vi "Frame Import UI.vi"(8 "error in":errorcluster) -> (0 "error out":errorcluster, 1 "Cancelled":bool, 2 "frame map out":map{string, T1}(c390), 3 "Currently Loaded file":path)   [LabVIEW 2020, in "FrameEditor.lvlib"]
doc: "This template is for the Queued Message Handler design pattern.\n\nThe Event Handling Loop generates messages based on user interface actions.\n\nThe Message Handling Loop processes messages generated by the Event Handling Loop, or by other messages. The messages are string values, so new messages can be added easily to the Message Cases case structure in the Message Handling Loop. Each message cluster can also provide an optional value for Message Data, which is a variant that can be converted to whatever message-specific data is required."
uses:
  FrameEditor.lvlib
  controls/frame_record_type.ctl
  <instrlib>/AIM GmbH/_AIM 664/_controls/queue_header_generic.ctl
  controls/UI Data.ctl
  controls/frame_file_entry.ctl
  controls/Type of Payload.ctl
  controls/Payload Record Type.ctl
  <instrlib>/AIM GmbH/_AIM 664/helpers/EthFrameManagement/controls/arinc664_mac_src_info.ctl
  <instrlib>/AIM GmbH/_AIM 664/helpers/EthFrameManagement/controls/arinc664_ip_src_info.ctl
  support/Message Queue/Enqueue Message (Single).vi
  <instrlib>/AIM GmbH/_AIM 664/helpers/EthFrameManagement/Create Payload (Constant).vi
  <instrlib>/AIM GmbH/_AIM 664/helpers/EthFrameManagement/Create Payload (Increment).vi
  <instrlib>/AIM GmbH/_AIM 664/helpers/EthFrameManagement/Create Payload (Random).vi
  <vilib>/Utility/error.llb/Error Cluster From Error Code.vi
  <vilib>/ErrorRing/Error Ring.xnode
  support/Message Queue/Message Queue.lvlib
  support/User Event - Stop/User Event - Stop.lvlib
  <instrlib>/AIM GmbH/_AIM 664/AIM664LV.lvlib
  <instrlib>/AIM GmbH/_AIM 664/helpers/EthFrameManagement/EthFrameManagement.lvlib
panel:
  in  "Frames":i32(listbox)
  out "Destination IP":string
  out "Source MAC":string
  out "Destination MAC":string
  out "Source IP":string
  in  "Partition ID":u8=1
  in  "Interface ID":u8=1 format="%.0b"
  in  "Location ID":u8=1
  in  "Side ID":u8=1
  in  "Domain ID":u8=1
  in  "Increment":u8=1 format="%.0x"
  in  "Start":u8=65 format="%02x"
  in  "Fill Value":u8=10 format="%02x"
  out "option":u32
  in  "Random Payload":bool
  in  "Increment Payload":bool
  in  "Fill Payload":bool
  in  "Bit Length":u16(ring) items=["Byte (8 bits)", "Word (16 bits)", "Long (32 bits)", "Quad (64 bits)"]
  in  "Clear Payload":bool
  in  "Frame ID":string="Frame1"
  in  "Payload Size":u32=17
  in  "Payload":u8[](array[numeric])=[0, 0, 0, 0, 0, 0, 0, 0, 0, 0, 0, 0, 0, 0, 0, 0, 0] format="%02x"
  in  "VL Id":u16=60
  in  "UDP Destination Port":u16=1
  in  "UDP Source Port":u16=1
  in  "Header Information":T3={"Inter Frame Gap"=0, "Packet Group Wait Time"=10000, "Payload Buffer Mode"=0, "Payload Generation Mode"=0, "Preamble Count"=7, "Skew"=0, "Net Select"=4, "Frame Start Mode"=1, "Physical Error Injection"=0, "Sequence Number Init"=65535, "Sequence Number Offset"=65535} {"Net Select" items=["FDX_TX_FRAME_DLY_A"=0, "FDX_TX_FRAME_DLY_B"=1, "FDX_TX_FRAME_BOTH "=3, "FDX_TX_FRAME_ONLY_A"=4, "FDX_TX_FRAME_ONLY_B "=5]; "Frame Start Mode" items=["FDX_TX_FRAME_START_IFG", "FDX_TX_FRAME_START_PGWT", "FDX_TX_FRAME_START_TRG"]; "Physical Error Injection" items=["FDX_TX_FRAME_ERR_OFF"=0, "FDX_TX_FRAME_ERR_CRC"=1, "FDX_TX_FRAME_ERR_ALI"=2, "FDX_TX_FRAME_ERR_PRE"=4, "FDX_TX_FRAME_ERR_PHY"=8]; "Sequence Number Init" items=["FDX_TX_FRAME_SEQ_INIT_AUTO"=65535]; "Sequence Number Offset" items=["FDX_TX_FRAME_SEQ_OFFS_AUTO "=65535]; "Payload Generation Mode" items=["FDX_TX_FRAME_PGM_USER"=0, "FDX_TX_FRAME_PGM_IP_PART"=1, "FDX_TX_FRAME_PGM_IP_FULL"=2, "FDX_TX_FRAME_PGM_IP_PART_TT"=10, "FDX_TX_FRAME_PGM_IP_FULL_TT"=20]; "Payload Buffer Mode" items=["FDX_TX_FRAME_PBM_STD", "FDX_TX_FRAME_PBM_MAC", "FDX_TX_FRAME_PBM_UDP"]}
  out "Payload Entry":string[][](table)
  out "Display Message":string
  in  "Convert":bool
  in  "Cancel":bool
  in  "Load":bool
  in  "Save":bool
  in  "Remove":bool
  in  "Add":bool
  in  "Exit":bool
  # "Auto-generate Payload"
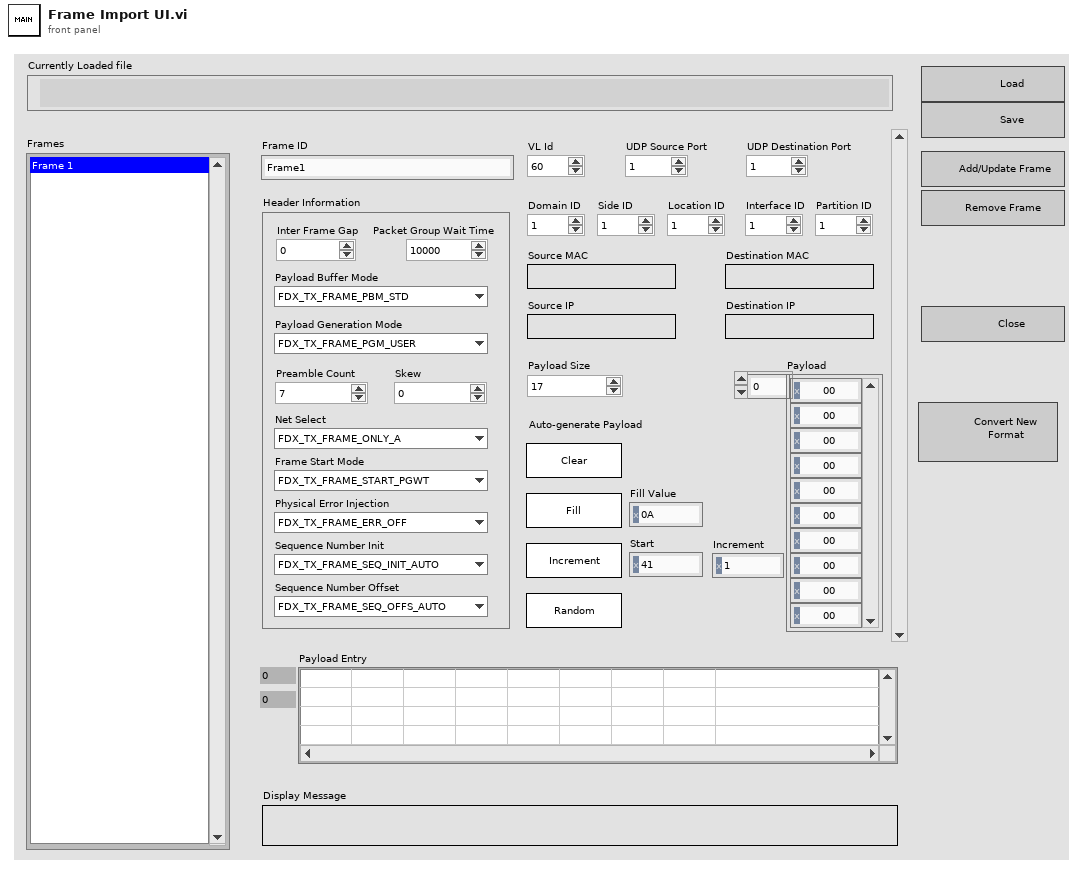
[diagram p1: front panel]
types:
  T1 = typedef "frame_record_type.ctl" = cluster{"HeaderInfo":T2, "Data":u8[]}
  T2 = typedef "AIM664LV.lvlib/queue_header_generic.ctl" = cluster{"InterFrameGap":u32, "PacketGroupWaitTime":u32, "PayloadBufferMode":u8, "PayloadGenerationMode":u8, "PreambleCount":u8, "Skew":u32, "NetSelect":u8, "FrameStartMode":u8, "PhysErrorInjection":u32, "SequenceNumberInit":u16, "SequenceNumberOffset":u16}
  T3 = cluster{"Inter Frame Gap":u32, "Packet Group Wait Time":u32, "Payload Buffer Mode":u8, "Payload Generation Mode":u8, "Preamble Count":u8, "Skew":u32, "Net Select":u8, "Frame Start Mode":u8, "Physical Error Injection":u32, "Sequence Number Init":u16, "Sequence Number Offset":u16}
  T4 = typedef "UI Data.ctl" = cluster{"changesPending":bool, "String <Replace Me>":string, "Numeric <Replace Me>":dbl, "Add":refnum<vi>, "Remove":refnum<vi>, "Data Display Ref":refnum<vi>, "Exit Button Ref":refnum<vi>, "Load":refnum<vi>, "Save":refnum<vi>, "Payload ID":refnum<vi>, "Type of Frame":refnum<vi>}
  T5 = typedef "FrameEditor.lvlib/Message Queue.lvlib/All Message Queues.ctl" = cluster{"UI":refnum<queue>}
  T6 = typedef "frame_file_entry.ctl" = cluster{"key":string, "value":T1}
  T7 = enum16{"open", "replace", "create", "open or create", "replace or create", "replace or create with confirmation"}
  T8 = typedef "Payload Record Type.ctl" = cluster{"Data":u8[], "Type of Frame":T9}
  T9 = typedef "Type of Payload.ctl" = u16
  T10 = typedef "EthFrameManagement.lvlib/arinc664_ip_src_info.ctl" = cluster{"domainID":u8, "sideID":u8, "locationID":u8, "partitionID":u8}
  T11 = typedef "EthFrameManagement.lvlib/arinc664_mac_src_info.ctl" = cluster{"domainID":u8, "sideID":u8, "locationID":u8, "interfaceID":u8}
  T12 = cluster{"Domain ID":u8, "Side ID":u8, "Location ID":u8, "Interface ID":u8, "Partition ID":u8}
  T13 = typedef "AIM664LV.lvlib/queue_data_full.ctl" = cluster{"domainID":u8, "sideID":u8, "locationID":u8, "interfaceID":u8, "partitionID":u8}
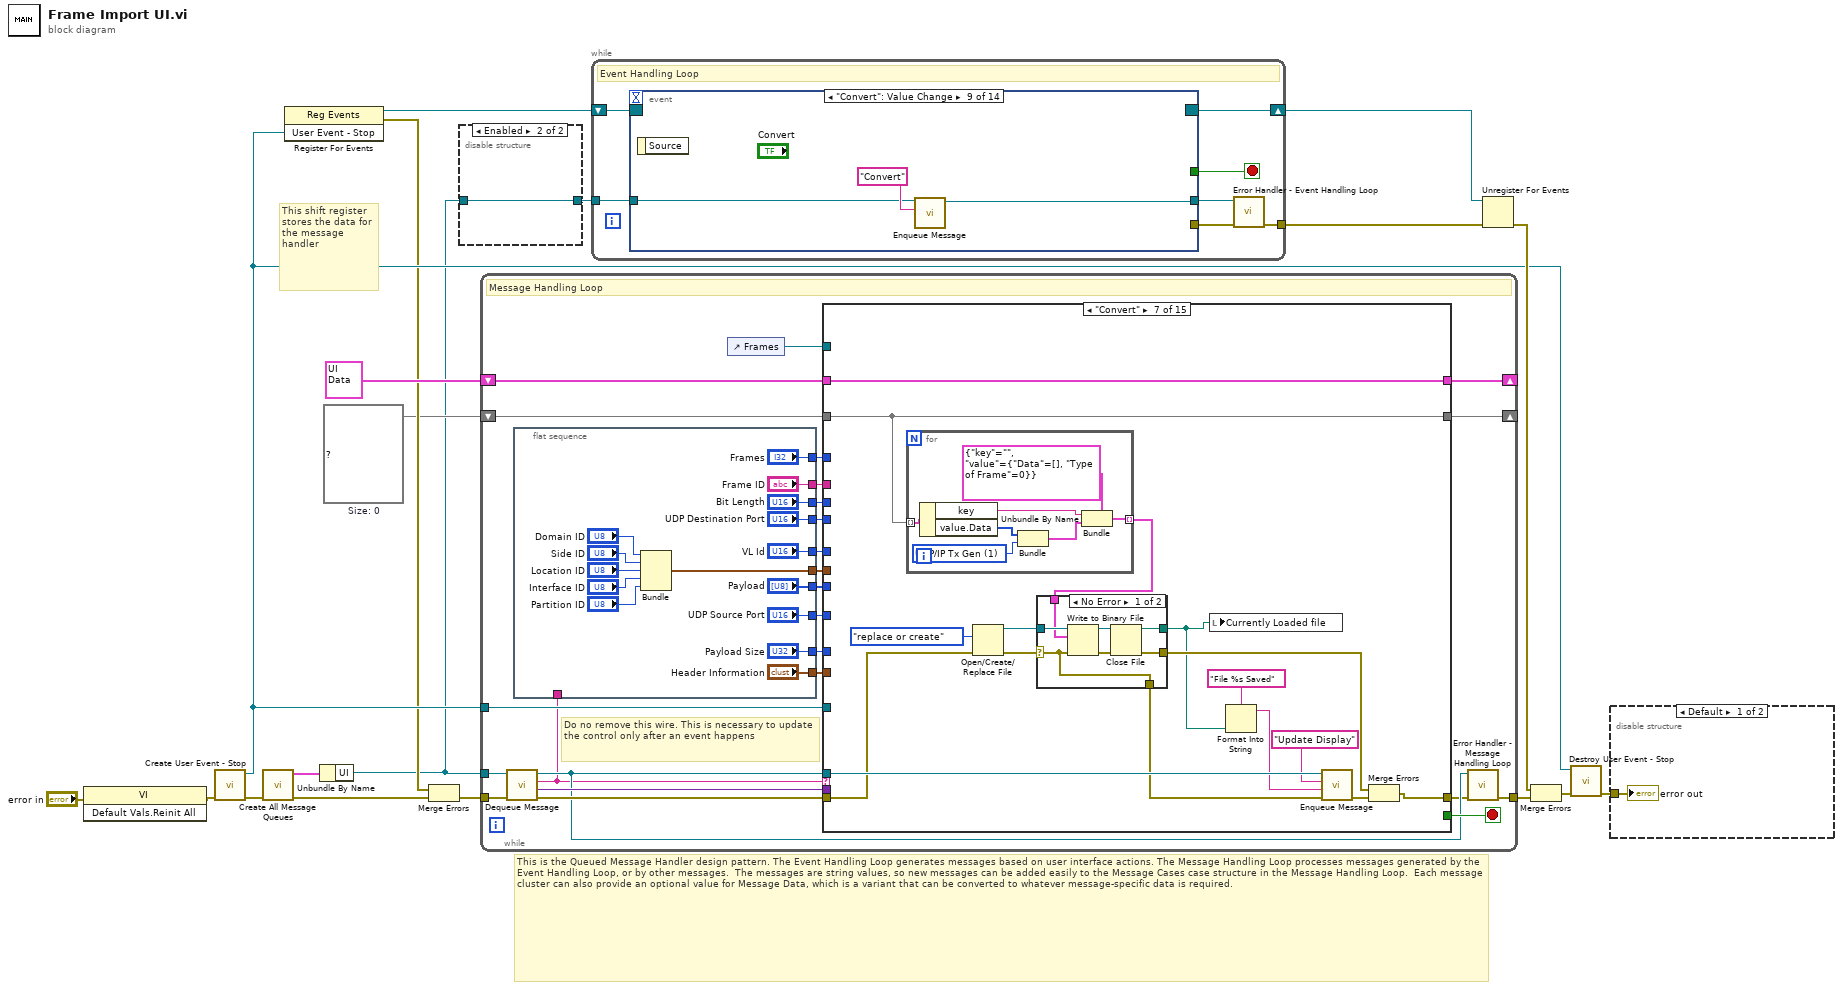
[diagram p0: block diagram]
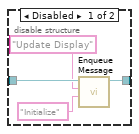
[diagram p2: hidden frame]
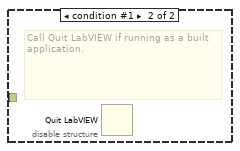
[diagram p3: hidden frame]
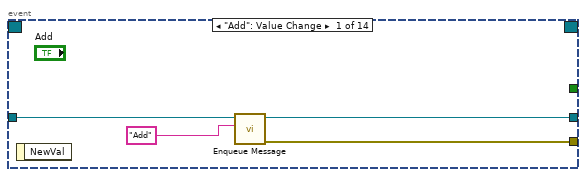
[diagram p4: hidden frame]
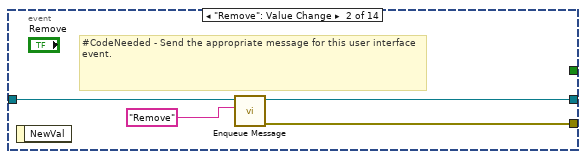
[diagram p5: hidden frame]
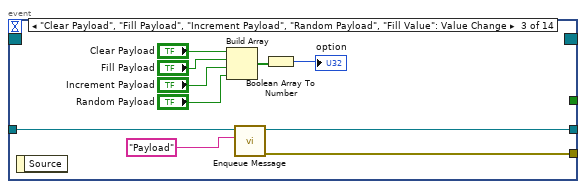
[diagram p6: hidden frame]
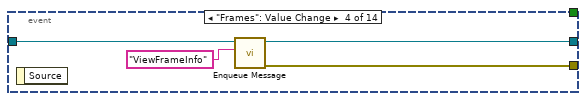
[diagram p7: hidden frame]
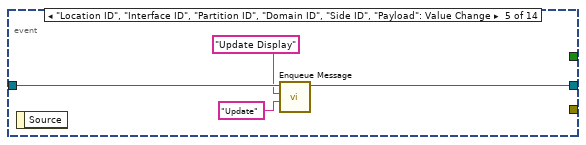
[diagram p8: hidden frame]
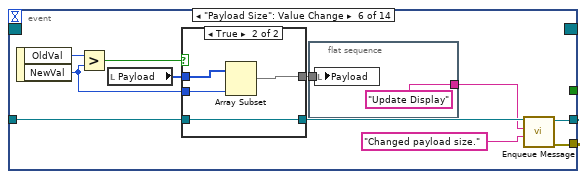
[diagram p9: hidden frame]
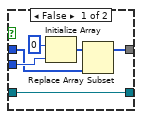
[diagram p10: hidden frame]
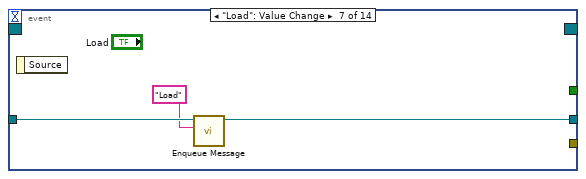
[diagram p11: hidden frame]
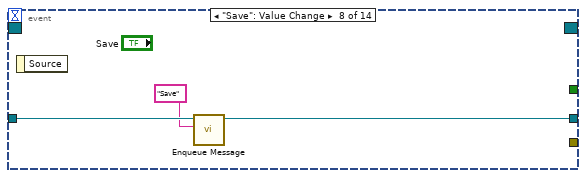
[diagram p12: hidden frame]
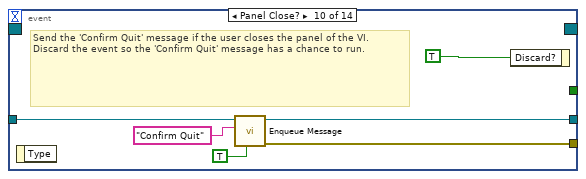
[diagram p13: hidden frame]
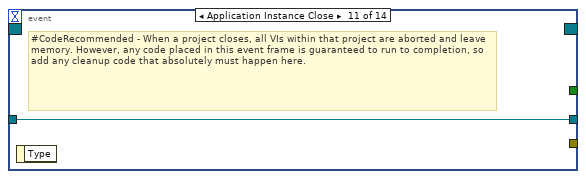
[diagram p14: hidden frame]
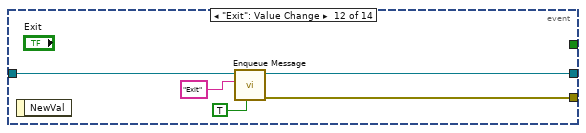
[diagram p15: hidden frame]
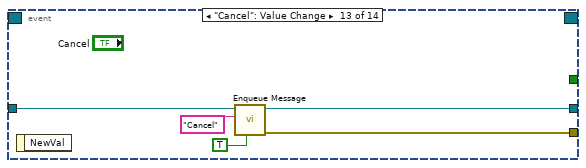
[diagram p16: hidden frame]
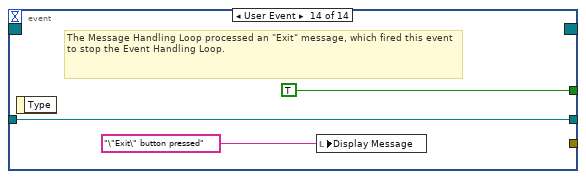
[diagram p17: hidden frame]
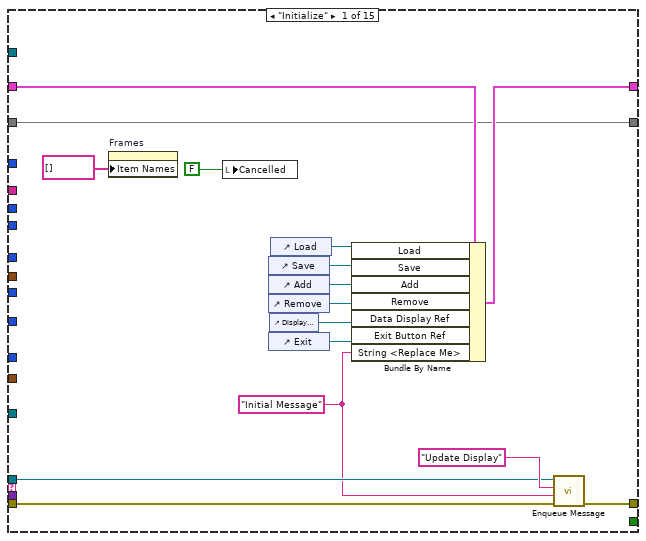
[diagram p18: hidden frame]
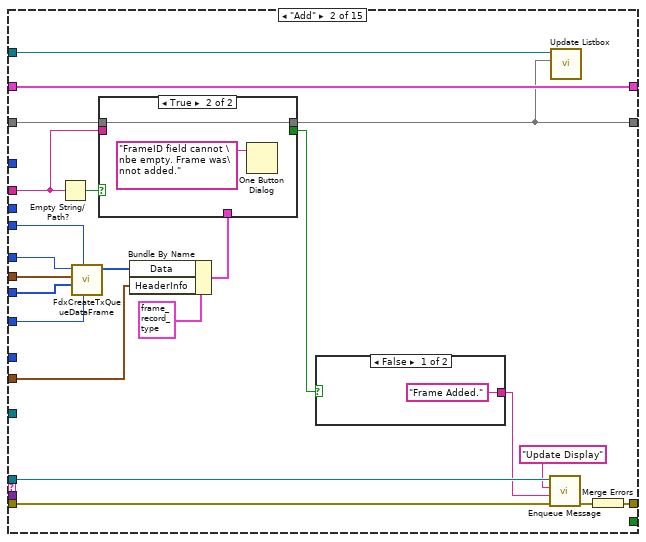
[diagram p19: hidden frame]
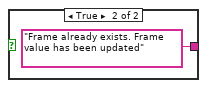
[diagram p20: hidden frame]
diagram:
  w5 = map{string, T1} {}  # Size: 0
  # "This is the Queued Message Handler design pattern. The Event Handling Loop generates messages based on user interface actions. The Message Handling Loop processes messages generated by the Event Handling Loop, or by other messages.  The messages are string values, so new messages can be added easily to the Message Cases case structure in the Message Handling Loop.  Each message cluster can also provide an optional value for Message Data, which is a variant that can be converted to whatever message-specific data is required."
  # "This shift register stores the data for the message handler"
  n1 = invoke class="VI" method="Default Vals.Reinit All"(error in="error in") -> (error out=w2:errorcluster)  [unwired: 2 in, 2 out]
  n2 = call "Create User Event - Stop.vi"("error in (no error)"=w2) -> ("error out"=w16:errorcluster, "User Event - Stop"=w8:refnum<user-event>)  [unwired: 9 in]
  n3 = call "Create All Message Queues.vi"("error in (no error)"=w16) -> ("error out"=w19:errorcluster, "Message Queues out"=w18:T5)  [unwired: 9 in]
  n4 = register-events(w8) -> (reference out=w9:refnum<event-registration>, error out=w6:errorcluster)  [unwired: 2 in]
  n5 = Unbundle By Name(w18) -> ("UI"=w4:refnum<queue>)
  n6 = Merge Errors(w6, w19) -> (w7:errorcluster)
  n7 = disable-structure shown="Enabled" {
    disable-tunnel: w4 -> [w23 w24]
    disable-tunnel: [w22 w24] -> w3
    frame Disabled {
      n8 = call-poly "Enqueue Message.vi"("Message Data"="Initialize" ("Message"), "Message"="Update Display", "Message Queue"=w23) -> ("dup Message Queue"=w22:refnum<queue>)  [unwired: 7 in, 1 out]
    }
    frame Enabled {
    }
  }
  n9 = while {
    tunnel: w4 -> [w42]
    shift-right: [w48] -> _
    shift-left: T4 {"changesPending"=FALSE, "String <Replace Me>"="", "Numeric <Replace Me>"=0.0, "Add"=refnum, "Remove"=refnum, "Data Display Ref"=refnum, "Exit Button Ref"=refnum, "Load"=refnum, "Save"=refnum, "Payload ID"=refnum, "Type of Frame"=refnum} ("Data Cluster") -> [w49]
    tunnel: w8 -> [w46]
    tunnel: w7 -> [w45]
    tunnel: [w40] -> w17
    shift-right: [w29] -> _
    shift-left: w5 -> [w31]
    stop <- w47 stop-if-true
    # "Do no remove this wire. This is necessary to update the control only after an event happens"
    # "Message Handling Loop"
    n10 = call "Dequeue Message.vi"("error in (no error)"=w45, "Message Queue"=w42) -> ("error out"=w44:errorcluster, "Message Data"=w43:variant, "Message"=w25:string, "dup Message Queue"=w41:refnum<queue>)  [unwired: 6 in]
    n11 = flat-sequence {
      tunnel: ["Payload Size"] -> w38
      tunnel: [w63] -> w37
      tunnel: ["VL Id"] -> w36
      tunnel: ["UDP Source Port"] -> w35
      tunnel: ["UDP Destination Port"] -> w34
      tunnel: ["Payload"] -> w33
      tunnel: ["Header Information"] -> w32
      tunnel: ["Frame ID"] -> w30
      tunnel: ["Frames"] -> w28
      tunnel: ["Bit Length"] -> w26
      tunnel: w25 -> [_]
      frame #0 {
        n12 = Bundle("Domain ID"="Domain ID", "Side ID"="Side ID", "Location ID"="Location ID", "Interface ID"="Interface ID", "Partition ID"="Partition ID") -> (w63:T12)  [unwired: 1 in]
      }
    }
    n13 = control-ref of="Frames"() -> (w27:refnum<vi>)
    n14 = case "Message Cases" shown="\"Convert\"" w25 {
      selector: w25 -> [_ _ _ _ _ _ _ _ _ _ _ _ _ _ w395]
      tunnel: w41 -> [w71 w98 w123 w162 w178 w213 w244 _ _ w328 _ w339 w380 w393 _]
      tunnel: w44 -> [w79 w100 w120 w164 w180 w211 w242 w302 w324 w332 w336 w342 w373 w386 _]
      tunnel: [w80 w101 w125 w165 w181 w215 w246 w303 w318 w330 w334 w347 w376 w389 w396] -> w39
      tunnel: w49 -> [w78 w102 w126 w166 w182 w216 w247 w304 w323 w331 w335 w348 w379 w392 w397]
      tunnel: [w77 w102 w126 w166 w182 w216 w247 w304 w323 w331 w335 w348 w379 w392 w397] -> w48
      tunnel: [_ _ _ _ _ _ _ _ _ _ _ _ TRUE TRUE _] -> w47
      tunnel: w43 -> [_ _ _ _ _ _ _ w301 w322 _ _ _ w370 w383 _]
      tunnel: w46 -> [_ _ _ _ _ _ _ _ _ _ _ _ w375 w388 _]
      tunnel: w38 -> [_ _ _ _ _ _ _ _ _ _ _ w345 _ _ _]
      tunnel: w37 -> [_ w95 _ _ _ _ _ w284 _ _ _ _ _ _ _]
      tunnel: w36 -> [_ w96 _ _ _ _ _ w285 _ _ _ _ _ _ _]
      tunnel: w35 -> [_ w92 _ _ _ _ _ _ _ _ _ _ _ _ _]
      tunnel: w34 -> [_ w94 _ _ _ _ _ _ _ _ _ _ _ _ _]
      tunnel: w33 -> [_ w93 _ _ _ _ _ w266 _ _ _ _ _ _ _]
      tunnel: w32 -> [_ w90 _ _ _ _ _ _ _ _ _ _ _ _ _]
      tunnel: w31 -> [w67 w85 w112 w159 w174 w210 w241 w269 w317 w325 w333 w346 w369 w382 w394]
      tunnel: w30 -> [_ w86 _ _ _ _ _ _ _ _ _ _ _ _ _]
      tunnel: [w67 w84 w117 w156 w174 w210 w241 w269 w317 w325 w333 w346 w369 w382 w394] -> w29
      tunnel: w28 -> [_ _ _ w152 w176 _ _ _ _ _ _ _ _ _ _]
      tunnel: w27 -> [_ w88 w121 w157 w175 _ _ w268 _ _ _ _ _ _ _]
      tunnel: w26 -> [_ _ _ _ _ _ _ w297 _ _ _ w344 _ _ _]
      frame "Initialize" {
        w70 = "Initial Message" ("Initial Message")
        # "Initialize - All initialization work should take place in this message, since other loops can potentially enqueue messages that execute immediately after this one."
        n15 = property on="Frames" class="LstBox (strict)"("Item Names"=string[] []) -> ()  [unwired: 2 in, 2 out]
        n16 = local write "Cancelled"(FALSE ("Cancel")) -> ()
        n17 = control-ref of="Save"() -> (w68:refnum<vi>)
        n18 = control-ref of="Add"() -> (w76:refnum<vi>)
        n19 = control-ref of="Remove"() -> (w75:refnum<vi>)
        n20 = control-ref of="Exit"() -> (w73:refnum<vi>)
        n21 = control-ref of="Display Message"() -> (w74:refnum<vi>)
        n22 = control-ref of="Load"() -> (w69:refnum<vi>)
        n23 = Bundle By Name(cluster=w78, "Load"=w69, "Save"=w68, "Add"=w76, "Remove"=w75, "Data Display Ref"=w74, "Exit Button Ref"=w73, "String <Replace Me>"=w70) -> (w77:T4)
        n24 = call-poly "Enqueue Message.vi"("error in (no error)"=w79, "Message Data"=w70, "Message"="Update Display", "Message Queue"=w71) -> ("error out"=w80:errorcluster)  [unwired: 6 in, 1 out]
      }
      frame "Add" {
        # "Something - Replace this message with functionality for your own application."
        n25 = Empty String/Path?(string/path=w86) -> (empty?=w87:bool)
        n26 = call <instrlib>:"FdxCreateTxQueueDataFrame.vi"("UDPsrcPort"=w92, "UDPdstPort"=w94, "Payload"=w93, "afdx configuration"=w95, "VL Id"=w96) -> ("Frame"=w89:u8[])  [unwired: 4 in, 2 out]
        n27 = Bundle By Name(cluster=T1 {"HeaderInfo"={"InterFrameGap"=0, "PacketGroupWaitTime"=10000, "PayloadBufferMode"=0, "PayloadGenerationMode"=0, "PreambleCount"=7, "Skew"=0, "NetSelect"=4, "FrameStartMode"=1, "PhysErrorInjection"=0, "SequenceNumberInit"=65535, "SequenceNumberOffset"=65535}, "Data"=[10]}, "Data"=w89, "HeaderInfo"=w90) -> (w83:T1)
        n28 = case shown="True" w87 {
          tunnel: w86 -> [w108 _]
          tunnel: w85 -> [w109 w110]
          tunnel: [w107 w110] -> w84
          tunnel: w83 -> [w106 _]
          tunnel: [w105 _] -> w82
          frame False {
            n29 = Insert Into Map(map in=w109, key=w108, value=w106) -> (map out=w107:map{string, T1}, key already included?=w105:bool)  [unwired: 1 out]
          }
          frame True {
            n30 = One Button Dialog(message="FrameID field cannot \nbe empty. Frame was\nnot added.") -> ()  [unwired: 1 in, 1 out]
          }
        }
        n31 = case shown="False" w82 {
          tunnel: ["Frame Added." ("format string") "Frame already exists. Frame value has been updated" ("format string")] -> w81
          frame False {
          }
          frame True {
          }
        }
        n32 = call-poly "Enqueue Message.vi"("error in (no error)"=w100, "Message Data"=w81, "Message"="Update Display", "Message Queue"=w98) -> ("error out"=w99:errorcluster)  [unwired: 6 in, 1 out]
        n33 = call "Update Listbox.vi"("frame map"=w84, "ListBox ref"=w88) -> ()  [unwired: 10 in]
        n34 = Merge Errors(w99) -> (w101:errorcluster)
      }
      frame "Load" {
        # "Something - Replace this message with functionality for your own application."
        n35 = Open/Create/Replace File(error in=w120) -> (refnum out=w118:refnum<file>, error out=w113:errorcluster)  [unwired: 5 in, 1 out]
        n36 = case shown="No Error" w113 {
          tunnel: w121 -> [w139 _]
          tunnel: [w128 _] -> w119
          tunnel: w118 -> [w138 _]
          tunnel: [w135 w151] -> w117
          tunnel: [w134 path "" ("path")] -> w115
          tunnel: w113 -> [w133 _]
          tunnel: ["File %s Loaded" ("format string") "Load Cancelled." ("format string")] -> w114
          tunnel: w112 -> [w127 w151]
          frame No Error {
            w137 = map{string, T1} {}  # Size: 0
            n37 = Read from Binary File(5:T6[] [] ("cluster"), 8:w133, 11:w138) -> (0:w131:errorcluster, 2:w136:T6[], 3:w130:refnum<file>)  [unwired: 3 in, 1 out]
            n38 = Close File(refnum=w130, error in=w131) -> (path=w134:path, error out=w128:errorcluster)
            n39 = case shown="No Error" w128 {
              tunnel: w137 -> [w142 _]
              tunnel: w136 -> [w141 _]
              tunnel: [w140 w148] -> w135
              tunnel: w127 -> [_ w148]
              frame No Error {
                n40 = for {
                  shift-right: [w146] -> w140
                  shift-left: w142 -> [w147]
                  tunnel: w141 -> [w145] mode=indexing
                  n41 = Unbundle By Name(w145) -> ("key"=w144:string, "value"=w143:T1)
                  n42 = Insert Into Map(map in=w147, key=w144, value=w143) -> (map out=w146:map{string, T1})  [unwired: 2 out]
                }
              }
              frame Error {
                # "Any error, we keep what we \nhad before."
              }
            }
            n43 = local write "Currently Loaded file"(w134) -> ()
            n44 = call "Update Listbox.vi"("frame map"=w135, "ListBox ref"=w139) -> ()  [unwired: 10 in]
          }
          frame Error {
          }
        }
        n45 = Format Into String(format string=w114, w115) -> (resulting string=w116:string)  [unwired: 2 in, 1 out]
        n46 = call-poly "Enqueue Message.vi"("error in (no error)"=w120, "Message Data"=w116, "Message"="Update Display", "Message Queue"=w123) -> ("error out"=w124:errorcluster)  [unwired: 6 in, 1 out]
        n47 = Merge Errors(w119, w124) -> (w125:errorcluster)
      }
      frame "Remove" {
        # "Something Else - Replace this message with functionality for your own application."
        n48 = invoke on="Frame ID" class="Str" method="Reinit To Default"() -> ()  [unwired: 3 in, 3 out]
        n49 = invoke on="UDP Destination Port" class="DigNum (strict)" method="Reinit To Default"() -> ()  [unwired: 3 in, 3 out]
        n50 = invoke on="VL Id" class="DigNum (strict)" method="Reinit To Default"() -> ()  [unwired: 3 in, 3 out]
        n51 = property on="Frames" class="LstBox (strict)"() -> ("Item Names"=w160:string[])  [unwired: 2 in, 2 out]
        n52 = Equal?(x=w152, y=-1) -> (x = y?=w154:bool)
        n53 = Index Array(array=w160, index=w152) -> (element=w158:string)
        n54 = case shown="False" w154 {
          tunnel: ["Frame removed." ("format string") "Frame was not selected, so no Frames were removed." ("format string")] -> w153
          frame False {
          }
          frame True {
          }
        }
        n55 = invoke on="UDP Source Port" class="DigNum (strict)" method="Reinit To Default"() -> ()  [unwired: 3 in, 3 out]
        n56 = invoke on="Payload" class="Arr (strict)" method="Reinit To Default"() -> ()  [unwired: 3 in, 3 out]
        n57 = invoke on="Payload Size" class="DigNum (strict)" method="Reinit To Default"() -> ()  [unwired: 3 in, 3 out]
        n58 = invoke on="Header Information" class="Clust (strict)" method="Reinit To Default"() -> ()  [unwired: 3 in, 3 out]
        n59 = Remove From Map(10:w158, 11:w159) -> (3:w156:map{string, T1})  [unwired: 2 out]
        n60 = call "Update Listbox.vi"("frame map"=w156, "ListBox ref"=w157) -> ()  [unwired: 10 in]
        n61 = call-poly "Enqueue Message.vi"("error in (no error)"=w164, "Message Data"=w153, "Message"="Update Display", "Message Queue"=w162) -> ("error out"=w163:errorcluster)  [unwired: 6 in, 1 out]
        n62 = Merge Errors(w163) -> (w165:errorcluster)
      }
      frame "ViewFrameInfo" {
        # "Something Else - Replace this message with functionality for your own application."
        n63 = property on="Frames" class="LstBox (strict)"() -> ("Item Names"=w177:string[])  [unwired: 2 in, 2 out]
        n64 = Index Array(array=w177, index=w176) -> (element=w169:string)
        n65 = Look In Map(map=w174, key=w169) -> (key not found?=w173:bool, value=w172:T1)  [unwired: 1 in]
        n66 = case shown="False" w173 {
          tunnel: w172 -> [w199 _]
          tunnel: [w197 "Frame not found"] -> w170
          tunnel: w169 -> [w190 _]
          frame False {
            n67 = Unbundle By Name(w199) -> ("HeaderInfo"=w196:T2, "Data"=w194:u8[])
            n68 = local write "Frame ID"(w190) -> ()
            n69 = local write "Header Information"(w196) -> ()
            n70 = call "Parse Raw Frame.vi"("Data"=w194, "HeaderInfo"=w196) -> ("UDPsrcPort"=w191:u16, "UDPdstPort"=w192:u16, "VL Id"=w193:u16, "Payload"=w184:u8[], "Frame Configuration"=w195:T13)  [unwired: 5 in]
            n71 = Format Into String(format string="Frame %s displayed", w190) -> (resulting string=w197:string)  [unwired: 2 in, 1 out]
            n72 = Unbundle(w195) -> ("domainID"=w189:u8, "sideID"=w185:u8, "locationID"=w188:u8, "interfaceID"=w186:u8, "partitionID"=w187:u8)
            n73 = Array Size(array=w184) -> (size(s)=w183:i32)
            n74 = local write "UDP Destination Port"(w192) -> ()
            n75 = local write "UDP Source Port"(w191) -> ()
            n76 = local write "Payload Size"(w183) -> ()
            n77 = local write "Location ID"(w188) -> ()
            n78 = local write "Interface ID"(w186) -> ()
            n79 = local write "Partition ID"(w187) -> ()
            n80 = local write "Domain ID"(w189) -> ()
            n81 = local write "Payload"(w184) -> ()
            n82 = local write "Side ID"(w185) -> ()
            n83 = local write "VL Id"(w193) -> ()
          }
          frame True {
          }
        }
        n84 = call "Update Listbox.vi"("frame map"=w174, "ListBox ref"=w175) -> ()  [unwired: 10 in]
        n85 = call-poly "Enqueue Message.vi"("error in (no error)"=w180, "Message Data"=w170, "Message"="Update Display", "Message Queue"=w178) -> ("error out"=w179:errorcluster)  [unwired: 6 in, 1 out]
        n86 = Merge Errors(w179) -> (w181:errorcluster)
      }
      frame "Save" {
        # "Something Else - Replace this message with functionality for your own application."
        n87 = for {
          tunnel: w210 -> [w231] mode=indexing
          tunnel: [w228] -> w207 mode=indexing
          n88 = Unbundle By Name(w231) -> ("key"=w230:string, "value"=w229:T1)
          n89 = Bundle(cluster=T6 {"key"="", "value"={"HeaderInfo"={"InterFrameGap"=0, "PacketGroupWaitTime"=0, "PayloadBufferMode"=0, "PayloadGenerationMode"=0, "PreambleCount"=0, "Skew"=0, "NetSelect"=0, "FrameStartMode"=0, "PhysErrorInjection"=0, "SequenceNumberInit"=0, "SequenceNumberOffset"=0}, "Data"=[]}}, "key"=w230, "value"=w229) -> (w228:T6)
        }
        n90 = Open/Create/Replace File(error in=w211, operation (0:open)=T7."replace or create") -> (refnum out=w209:refnum<file>, error out=w202:errorcluster)  [unwired: 4 in, 1 out]
        n91 = case shown="No Error" w202 {
          selector: w202 -> [w217 w225]
          tunnel: w209 -> [w223 _]
          tunnel: [w220 w224] -> w208
          tunnel: w207 -> [w219 _]
          tunnel: [w218 _] -> w204
          tunnel: [w217 w224] -> w201
          frame No Error {
            n92 = Write to Binary File(file (use dialog)=w223, data=w219, error in=w217) -> (refnum out=w221:refnum<file>, error out=w222:errorcluster)  [unwired: 3 in, 1 out]
            n93 = Close File(refnum=w221, error in=w222) -> (path=w218:path, error out=w220:errorcluster)
          }
          frame Error {
            n94 = call <vilib>:"Clear Errors.vi"("error in (no error)"=w225, "specific error code to clear (0: all)"=43) -> ("error out"=w224:errorcluster)  [unwired: 4 in, 1 out]
          }
        }
        "Currently Loaded file" <- w204
        n95 = Format Into String(format string="File %s Saved", w204) -> (resulting string=w206:string)  [unwired: 2 in, 1 out]
        n96 = call-poly "Enqueue Message.vi"("error in (no error)"=w201, "Message Data"=w206, "Message"="Update Display", "Message Queue"=w213) -> ("error out"=w214:errorcluster)  [unwired: 6 in, 1 out]
        n97 = Merge Errors(w208, w214) -> (w215:errorcluster)
      }
      frame "Convert" {
        # "Something Else - Replace this message with functionality for your own application."
        n98 = for {
          tunnel: w241 -> [w264] mode=indexing
          tunnel: [w259] -> w238 mode=indexing
          w263 = T9 1 items=["Raw Frame", "UDP/IP Tx Gen", "Tx UDP"] ("Type of Frame")
          n99 = Unbundle By Name(w264) -> ("key"=w260:string, "value.Data"=w262:u8[])
          n100 = Bundle("Data"=w262, "Type of Frame"=w263) -> (w261:cluster{"Data":u8[], "Type of Frame":T9})  [unwired: 1 in]
          n101 = Bundle(cluster=cluster{"key":string, "value":T8} {"key"="", "value"={"Data"=[], "Type of Frame"=0}}, "key"=w260, "value"=w261) -> (w259:cluster{"key":string, "value":T8})
        }
        n102 = Open/Create/Replace File(error in=w242, operation (0:open)=T7."replace or create") -> (refnum out=w240:refnum<file>, error out=w234:errorcluster)  [unwired: 4 in, 1 out]
        n103 = case shown="No Error" w234 {
          selector: w234 -> [w248 w256]
          tunnel: w240 -> [w254 _]
          tunnel: [w251 w255] -> w239
          tunnel: w238 -> [w250 _]
          tunnel: [w249 _] -> w232
          tunnel: [w248 w255] -> w233
          frame No Error {
            n104 = Write to Binary File(file (use dialog)=w254, data=w250, error in=w248) -> (refnum out=w252:refnum<file>, error out=w253:errorcluster)  [unwired: 3 in, 1 out]
            n105 = Close File(refnum=w252, error in=w253) -> (path=w249:path, error out=w251:errorcluster)
          }
          frame Error {
            n106 = call <vilib>:"Clear Errors.vi"("error in (no error)"=w256, "specific error code to clear (0: all)"=43) -> ("error out"=w255:errorcluster)  [unwired: 4 in, 1 out]
          }
        }
        n107 = local write "Currently Loaded file"(w232) -> ()
        n108 = Format Into String(format string="File %s Saved", w232) -> (resulting string=w237:string)  [unwired: 2 in, 1 out]
        n109 = call-poly "Enqueue Message.vi"("error in (no error)"=w233, "Message Data"=w237, "Message"="Update Display", "Message Queue"=w244) -> ("error out"=w245:errorcluster)  [unwired: 6 in, 1 out]
        n110 = Merge Errors(w239, w245) -> (w246:errorcluster)
      }
      frame "Update Display" {
        # "Update Display - Convert the message data to a string to display in the Data Display indicator."
        n111 = Increment(x=w297) -> (x+1=w295:u16)
        n112 = Multiply(x=w295, y=u16 8) -> (x*y=w265:u16)
        n113 = Variant To Data(error in=w302, type="", Variant=w301) -> (data=→"Display Message":string, error out=w299:errorcluster)
        n114 = call "Convert Non-visible Char to Visible Char.vi"("bytes per row"=w265, "data"=w266) -> ("data table"=→"Payload Entry":string[][])  [unwired: 7 in, 2 out]
        n115 = Unbundle By Name(w284) -> ("Domain ID"=w289:u8, "Side ID"=w288:u8, "Location ID"=w287:u8, "Interface ID"=w292:u8, "Partition ID"=w286:u8)
        n116 = Bundle By Name(cluster=T11 {"domainID"=0, "sideID"=0, "locationID"=0, "interfaceID"=1} ("Source Info"), "domainID"=w289, "sideID"=w288, "locationID"=w287, "interfaceID"=w292) -> (w293:T11)
        n117 = Bundle By Name(cluster=T10 {"domainID"=0, "sideID"=0, "locationID"=0, "partitionID"=1} ("Source Info"), "domainID"=w289, "sideID"=w288, "locationID"=w287, "partitionID"=w286) -> (w290:T10)
        n118 = call <instrlib>:"Create ARINC-664 IP (Dest).vi"("VL"=w285) -> ("ip string"=→"Destination IP":string)  [unwired: 8 in, 2 out]
        n119 = call <instrlib>:"Create ARINC-664 MAC (Dest).vi"("VL Id"=w285) -> ("MAC-src"=w279:u8[])  [unwired: 9 in, 1 out]
        n120 = for {
          tunnel: w279 -> [w310] mode=indexing
          shift-right: [w306] -> w270
          shift-left: "" -> [w305]
          n121 = Number To Hexadecimal String(1:i16 2 ("width (-)"), 2:w310) -> (0:w308:string)
          n122 = Concatenate Strings(w305, w308, ":" ("string")) -> (w306:string)
        }
        n123 = call <instrlib>:"Create ARINC-664 MAC (Source).vi"("Source Info"=w293) -> ("MAC-src"=w281:u8[])  [unwired: 9 in, 1 out]
        n124 = call <instrlib>:"Create ARINC-664 IP (Source).vi"("Source Info"=w290) -> ("ip address"=→"Source IP":string)  [unwired: 9 in, 1 out]
        n125 = for {
          tunnel: w281 -> [w316] mode=indexing
          shift-right: [w312] -> w276
          shift-left: "" -> [w311]
          n126 = Number To Hexadecimal String(1:i16 2 ("width (-)"), 2:w316) -> (0:w314:string)
          n127 = Concatenate Strings(w311, w314, ":" ("string")) -> (w312:string)
        }
        n128 = call "Update Listbox.vi"("frame map"=w269, "ListBox ref"=w268) -> ()  [unwired: 10 in]
        n129 = String Length(string=w270) -> (length=w272:i32)
        n130 = String Length(string=w276) -> (length=w275:i32)
        n131 = Decrement(x=w272) -> (x-1=w273:i32)
        n132 = String Subset(string=w270, length (rest)=w273) -> (substring=→"Destination MAC":string)  [unwired: 1 in]
        n133 = Merge Errors(w299) -> (w303:errorcluster)
        n134 = Decrement(x=w275) -> (x-1=w274:i32)
        n135 = String Subset(string=w276, length (rest)=w274) -> (substring=→"Source MAC":string)  [unwired: 1 in]
      }
      frame "Error" {
        # "#CodeRecommended - If you ever change the name of this \"Error\" message, you'll need to update the name in the Check Loop Error.vi as well."
        # "#CodeRecommended - Consider creating a system for logging errors in some way. These errors are for notification purposes only. Handling of specific errors should be performed in the message frames that generated the error."
        # "Error - Display an error dialog. This message is sent by the \"Error Handler\" VIs at the end of other loops in this application."
        n136 = Variant To Data(error in=w324, type=errorcluster {"status"=FALSE, "code"=0, "source"=""} ("error constant"), Variant=w322) -> (data=w320:errorcluster, error out=w319:errorcluster)
        n137 = call <vilib>:"Simple Error Handler.vi"("error in (no error)"=w320) -> ()  [unwired: 4 in, 5 out]
        n138 = Merge Errors(w319) -> (w318:errorcluster)
      }
      frame "Confirm Quit" {
        # "#CodeNeeded - If you want to provide an \"Are you sure\" dialog (or some other notification) before the application exits, place that code here. This message is typically sent from a Panel Close? event."
        # "Confirm Quit - Message that can confirm whether or not the user wants to exit the application."
        n139 = call-poly "Enqueue Message.vi"("Priority Message? (F)"=TRUE, "error in (no error)"=w332, "Message"="Exit", "Message Queue"=w328) -> ("error out"=w329:errorcluster)  [unwired: 6 in, 1 out]
        n140 = Merge Errors(w329) -> (w330:errorcluster)
      }
      frame "---Copy This Frame---" {
        # "Duplicate this frame when creating new messages.  Change this comment in the duplicated frame to describe this message."
        n141 = Merge Errors(w336) -> (w334:errorcluster)
      }
      frame "Payload" {
        # "Duplicate this frame when creating new messages.  Change this comment in the duplicated frame to describe this message."
        n142 = local read "option"() -> (w343:u32)
        n143 = case shown="1" w343 {
          tunnel: w345 -> [_ w353 w358 w362 w367]
          tunnel: w344 -> [_ w352 w357 w363 w366]
          tunnel: [_ w349 w354 w359 w365] -> w337
          frame Default {
          }
          frame 1 {
            n144 = call-poly <instrlib>:"Create Payload.vi"("Bit Length"=w352, "Value"=u64 0, "Length"=w353) -> ("error out"=w349:errorcluster, "Payload (U8)"=w351:u8[])  [unwired: 6 in, 1 out]
            n145 = local write "Payload"(w351) -> ()
          }
          frame 2 {
            n146 = call-poly <instrlib>:"Create Payload.vi"("Bit Length"=w357, "Value"="Fill Value", "Length"=w358) -> ("error out"=w354:errorcluster, "Payload (U8)"=w356:u8[])  [unwired: 6 in, 1 out]
            n147 = local write "Payload"(w356) -> ()
          }
          frame 4 {
            n148 = call-poly <instrlib>:"Create Payload.vi"("Bit Length"=w363, "Interval"="Increment", "Start Value"="Start", "Length"=w362) -> ("error out"=w359:errorcluster, "Payload (U8)"=w364:u8[])  [unwired: 5 in, 1 out]
            n149 = local write "Payload"(w364) -> ()
          }
          frame 8 {
            n150 = call-poly <instrlib>:"Create Payload.vi"("Bit Length"=w366, "Length"=w367) -> ("error out"=w365:errorcluster, "Payload (U8)"=w368:u8[])  [unwired: 7 in, 1 out]
            n151 = local write "Payload"(w368) -> ()
          }
        }
        n152 = call <vilib>:"Clear Errors.vi"("error in (no error)"=w337) -> ()  [unwired: 5 in, 2 out]
        n153 = call-poly "Enqueue Message.vi"("error in (no error)"=w342, "Message Data"="Created payload" ("Message"), "Message"="Update Display", "Message Queue"=w339) -> ("error out"=w341:errorcluster)  [unwired: 6 in, 1 out]
        n154 = Merge Errors(w341) -> (w347:errorcluster)
      }
      frame "Exit" {
        # "Stop the VI"
        # "Release the message queue reference"
        # "#CodeNeeded - Add any required cleanup code here. Note that if 'Exit' was called as a result of an error, an error dialog will be displayed. Add any custom error handling for an 'Exit' condition here as well."
        # "Exit - Exit the application."
        n155 = Variant To Data(type=errorcluster {"status"=FALSE, "code"=0, "source"=""} ("error constant"), Variant=w370) -> (data=w371:errorcluster)  [unwired: 1 in, 1 out]
        n156 = call <vilib>:"Simple Error Handler.vi"("error in (no error)"=w371) -> ()  [unwired: 4 in, 5 out]
        n157 = call "Fire User Event - Stop.vi"("User Event - Stop"=w375) -> ("error out"=w374:errorcluster)  [unwired: 10 in]
        n158 = Release Queue(queue=w380, error in (no error)=w373) -> (error out=w377:errorcluster)  [unwired: 1 in, 2 out]
        n159 = Merge Errors(w374, w377) -> (w376:errorcluster)
        "frame map out" <- w369
      }
      frame "Cancel" {
        # "Stop the VI"
        # "Release the message queue reference"
        # "#CodeNeeded - Add any required cleanup code here. Note that if 'Exit' was called as a result of an error, an error dialog will be displayed. Add any custom error handling for an 'Exit' condition here as well."
        # "Exit - Exit the application."
        n160 = Variant To Data(type=errorcluster {"status"=FALSE, "code"=0, "source"=""} ("error constant"), Variant=w383) -> (data=w384:errorcluster)  [unwired: 1 in, 1 out]
        n161 = call <vilib>:"Simple Error Handler.vi"("error in (no error)"=w384) -> ()  [unwired: 4 in, 5 out]
        n162 = call "Fire User Event - Stop.vi"("User Event - Stop"=w388) -> ("error out"=w387:errorcluster)  [unwired: 10 in]
        n163 = Release Queue(queue=w393, error in (no error)=w386) -> (error out=w390:errorcluster)  [unwired: 1 in, 2 out]
        n164 = Merge Errors(w387, w390) -> (w389:errorcluster)
        "Cancelled" <- TRUE ("Cancelled")
      }
      frame Default {
        # "'Default' case only runs if there is a message that isn't defined in any of the other cases.  Output a programming error."
        n165 = xnode "Error Ring"("parameter 0"=w395) -> ("error out"=w396:errorcluster)
      }
    }
    n166 = call "Error Handler - Message Handling Loop.vi"("error in (no error)"=w39, "Message Queue"=w41) -> ("dup error in"=w40:errorcluster)  [unwired: 8 in, 1 out]
  }
  n167 = while {
    tunnel: w3 -> [w411]
    shift-right: [w409] -> w13
    shift-left: w9 -> [w410]
    tunnel: [w405] -> w10
    stop <- w407 stop-if-true
    # "Event Handling Loop"
    n168 = event shown="[8] \"Convert\": Value Change" {
      selector: w410 -> [_ _ _ _ _ _ _ _ _ _ _ _ _ _]
      dyn-events: [_ _ _ _ _ _ _ _ _ _ _ _ _ _] -> w409
      timeout: _ -> [_ _ _ _ _ _ _ _ _ _ _ _ _ _]
      tunnel: [_ _ _ _ _ _ _ _ _ _ _ _ _ TRUE ("Discard?")] -> w407
      tunnel: w411 -> [w415 w419 w429 w433 w437 w441 w463 w466 w468 w474 w476 w481 w486 w489]
      tunnel: [w412 w416 w426 w430 _ w447 _ _ _ w473 _ w480 w485 _] -> w408
      tunnel: [w414 w418 w428 w432 w436 w446 w462 w465 w467 w472 w476 w479 w484 w489] -> w406
      event "Add": Value Change {
        n169 = event-data() -> ()  [unwired: 1 in, 1 out]
        n170 = call-poly "Enqueue Message.vi"("Message"="Add", "Message Queue"=w415) -> ("error out"=w412:errorcluster, "dup Message Queue"=w414:refnum<queue>)  [unwired: 8 in]
      }
      event "Remove": Value Change {
        # "#CodeNeeded - Send the appropriate message for this user interface event."
        n171 = event-data() -> ()  [unwired: 1 in, 1 out]
        n172 = call-poly "Enqueue Message.vi"("Message"="Remove", "Message Queue"=w419) -> ("error out"=w416:errorcluster, "dup Message Queue"=w418:refnum<queue>)  [unwired: 8 in]
      }
      event "Clear Payload", "Fill Payload", "Increment Payload", "Random Payload", "Fill Value": Value Change {
        n173 = event-data() -> ()  [unwired: 1 in, 1 out]
        n174 = Build Array("Clear Payload", "Fill Payload", "Increment Payload", "Random Payload") -> (w421:bool[])
        n175 = call-poly "Enqueue Message.vi"("Message"="Payload", "Message Queue"=w429) -> ("error out"=w426:errorcluster, "dup Message Queue"=w428:refnum<queue>)  [unwired: 8 in]
        n176 = Boolean Array To Number(Boolean array=w421) -> (number=→"option":u32)
      }
      event "Frames": Value Change {
        n177 = event-data() -> ()  [unwired: 1 in, 1 out]
        n178 = call-poly "Enqueue Message.vi"("Message"="ViewFrameInfo", "Message Queue"=w433) -> ("error out"=w430:errorcluster, "dup Message Queue"=w432:refnum<queue>)  [unwired: 8 in]
      }
      event "Location ID", "Interface ID", "Partition ID", "Domain ID", "Side ID", "Payload": Value Change {
        n179 = event-data() -> ()  [unwired: 1 in, 1 out]
        n180 = call-poly "Enqueue Message.vi"("Message Data"="Update" ("Message"), "Message"="Update Display", "Message Queue"=w437) -> ("dup Message Queue"=w436:refnum<queue>)  [unwired: 7 in, 1 out]
      }
      event "Payload Size": Value Change {
        n181 = event-data() -> ("OldVal"=w444:u32, "NewVal"=w442:u32)  [unwired: 1 in]
        n182 = Greater?(x=w444, y=w442) -> (0:w443:bool)
        n183 = local read "Payload"() -> (w448:u8[])
        n184 = case shown="True" w443 {
          tunnel: w448 -> [w453 w460]
          tunnel: [w454 w459] -> w445
          tunnel: w442 -> [w456 w458]
          tunnel: w441 -> [w451 w457]
          tunnel: [w451 w457] -> w440
          frame False {
            n185 = Initialize Array(u8 0 ("new element/subarray"), w456) -> (w452:u8[])
            n186 = Replace Array Subset(array=w452, new element=w453) -> (w454:u8[])  [unwired: 1 in]
          }
          frame True {
            n187 = Array Subset(array=w460, length=w458) -> (w459:u8[])  [unwired: 1 in]
          }
        }
        n188 = flat-sequence {
          tunnel: ["Update Display" ("Message")] -> w439
          tunnel: w445 -> [w449]
          frame #0 {
            n189 = local write "Payload"(w449) -> ()
          }
        }
        n190 = call-poly "Enqueue Message.vi"("Message Data"="Changed payload size." ("Message"), "Message"=w439, "Message Queue"=w440) -> ("error out"=w447:errorcluster, "dup Message Queue"=w446:refnum<queue>)  [unwired: 7 in]
      }
      event "Load": Value Change {
        n191 = event-data() -> ()  [unwired: 1 in, 1 out]
        n192 = call-poly "Enqueue Message.vi"("Message"="Load", "Message Queue"=w463) -> ("dup Message Queue"=w462:refnum<queue>)  [unwired: 8 in, 1 out]
      }
      event "Save": Value Change {
        n193 = event-data() -> ()  [unwired: 1 in, 1 out]
        n194 = call-poly "Enqueue Message.vi"("Message"="Save", "Message Queue"=w466) -> ("dup Message Queue"=w465:refnum<queue>)  [unwired: 8 in, 1 out]
      }
      event "Convert": Value Change {
        n195 = event-data() -> ()  [unwired: 1 in, 1 out]
        n196 = call-poly "Enqueue Message.vi"("Message"="Convert", "Message Queue"=w468) -> ("dup Message Queue"=w467:refnum<queue>)  [unwired: 8 in, 1 out]
      }
      event Panel Close? {
        # "Send the 'Confirm Quit' message if the user closes the panel of the VI. Discard the event so the 'Confirm Quit' message has a chance to run."
        n197 = event-data() -> ()  [unwired: 1 in, 1 out]
        n198 = call-poly "Enqueue Message.vi"("Priority Message? (F)"=TRUE, "Message"="Confirm Quit", "Message Queue"=w474) -> ("error out"=w473:errorcluster, "dup Message Queue"=w472:refnum<queue>)  [unwired: 7 in]
        n199 = event-data("Discard?"=TRUE) -> ()  [unwired: 1 in, 1 out]
      }
      event Application Instance Close {
        # "#CodeRecommended - When a project closes, all VIs within that project are aborted and leave memory. However, any code placed in this event frame is guaranteed to run to completion, so add any cleanup code that absolutely must happen here."
        n200 = event-data() -> ()  [unwired: 1 in, 1 out]
      }
      event "Exit": Value Change {
        n201 = event-data() -> ()  [unwired: 1 in, 1 out]
        n202 = call-poly "Enqueue Message.vi"("Priority Message? (F)"=TRUE, "Message"="Exit", "Message Queue"=w481) -> ("error out"=w480:errorcluster, "dup Message Queue"=w479:refnum<queue>)  [unwired: 7 in]
      }
      event "Cancel": Value Change {
        n203 = event-data() -> ()  [unwired: 1 in, 1 out]
        n204 = call-poly "Enqueue Message.vi"("Priority Message? (F)"=TRUE, "Message"="Cancel", "Message Queue"=w486) -> ("error out"=w485:errorcluster, "dup Message Queue"=w484:refnum<queue>)  [unwired: 7 in]
      }
      event User Event {
        # "The Message Handling Loop processed an \"Exit\" message, which fired this event to stop the Event Handling Loop."
        n205 = event-data() -> ()  [unwired: 1 in, 1 out]
        n206 = local write "Display Message"("\"Exit\" button pressed" ("VI Stopped")) -> ()
      }
    }
    n207 = call "Error Handler - Event Handling Loop.vi"("error in (no error)"=w408, "Message Queue"=w406) -> ("dup error in"=w405:errorcluster)  [unwired: 8 in, 1 out]
  }
  n208 = Unregister For Events(event registration refnum=w13, error in=w10) -> (error out=w14:errorcluster)
  n209 = Merge Errors(w14, w17) -> (w15:errorcluster)
  n210 = call "Destroy User Event - Stop.vi"("error in (no error)"=w15, "User Event - Stop"=w8) -> ("error out"=w11:errorcluster)  [unwired: 9 in]
  n211 = disable-structure shown="Default" {
    disable-tunnel: w11 -> [w490 _]
    frame condition #0 (active) {
      "error out" <- w490
    }
    frame condition #1 {
      # "Call Quit LabVIEW if running as a built application."
      n212 = Quit LabVIEW() -> ()  [unwired: 1 in]
    }
  }
